vi "getAxisSignalQuality.vi"(0 "connection ID":refnum<k5>, 1 "axis":i32, 5 "error":errorcluster) -> (14 "connection ID out":refnum<k5>, 15 "axis_out":i32, 16 "contrast":i32, 17 "baseline":i32, 19 "error out":errorcluster)   [LabVIEW 2016, in "sen_api.lvlib"]
doc: "This function can be used to monitor the signal contrast (peak-to-peak of the basic interference signal amplitude) and the baseline (its offset) during a running measurement."
uses:
  sen_api.lvlib
panel:
  out "jsonRespIn":string
  out "JSON-response":string="{\"jsonrpc\":\"2.0\",\"method\":\"\",\"params\":[5,1.245,true,\"name\"],\"id\":\"1\"}"
  out "JSON request":string
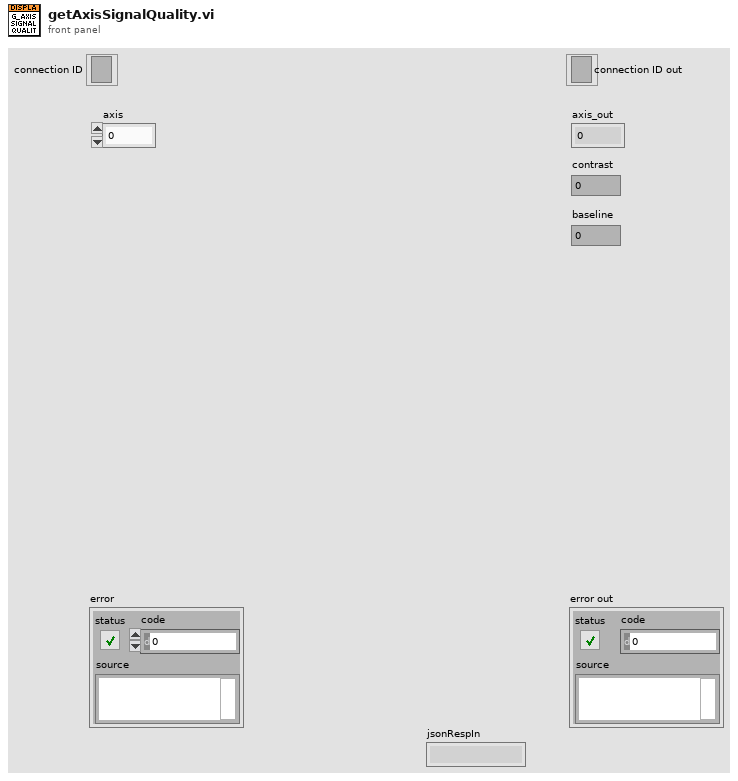
[diagram p1: front panel]
types:
  T1 = cluster{"jsonrpc":string, "method":string, "params":string[], "id":string, "api":i32, "pid":string}
  T2 = enum16{"Standard", "Buffered", "CRLF", "Immediate"}
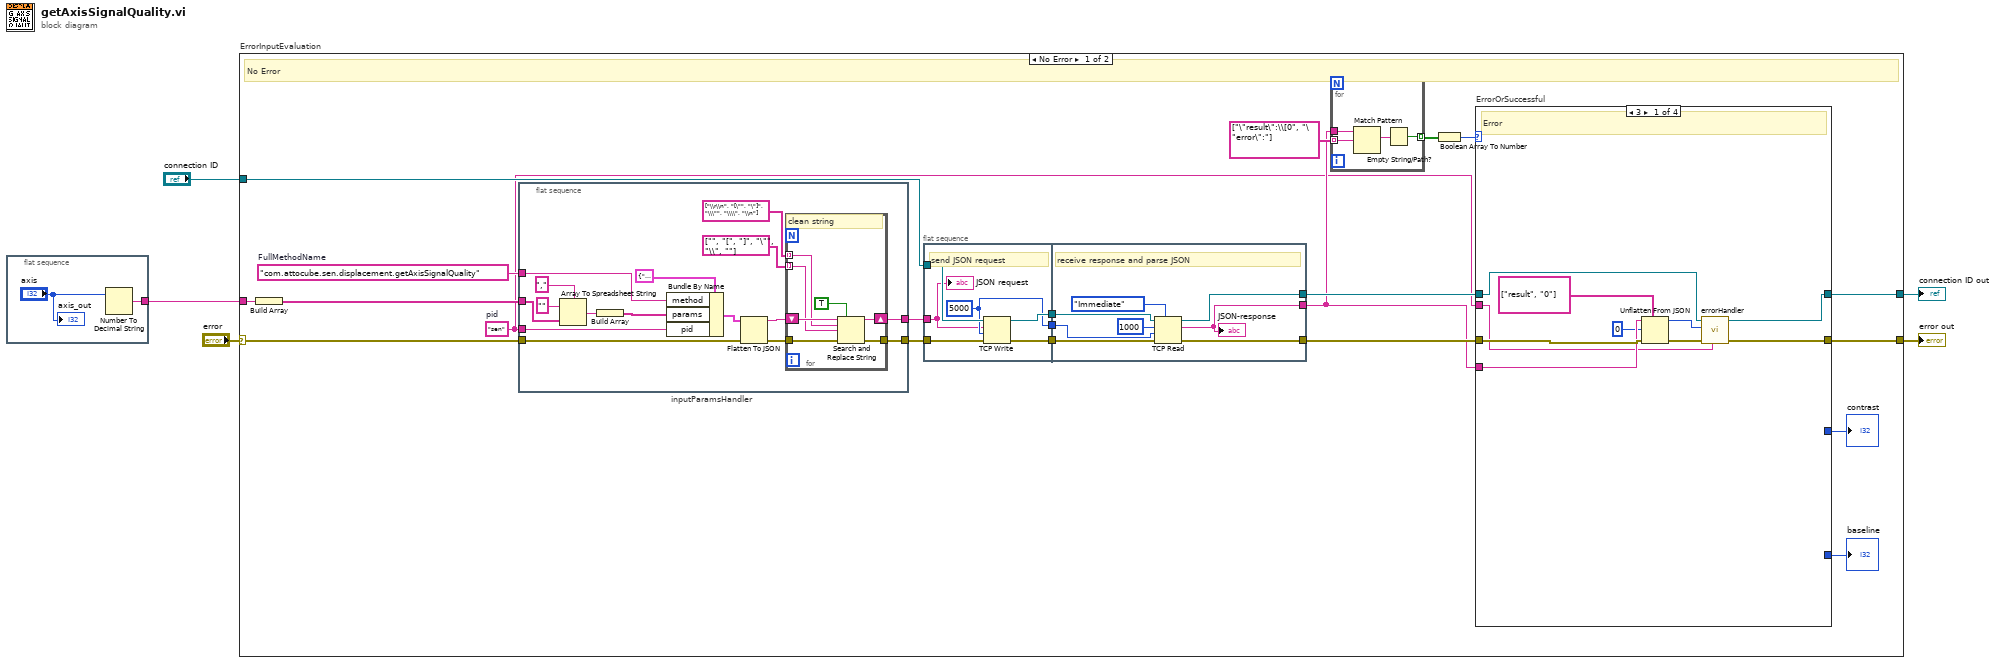
[diagram p0: block diagram]
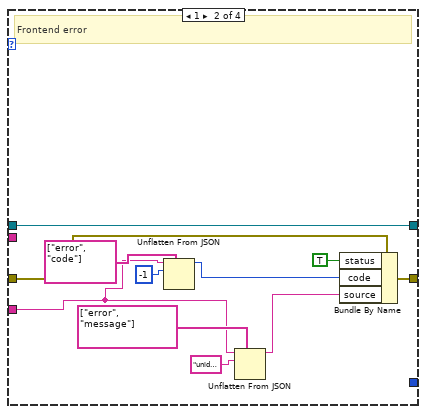
[diagram p2: hidden frame]
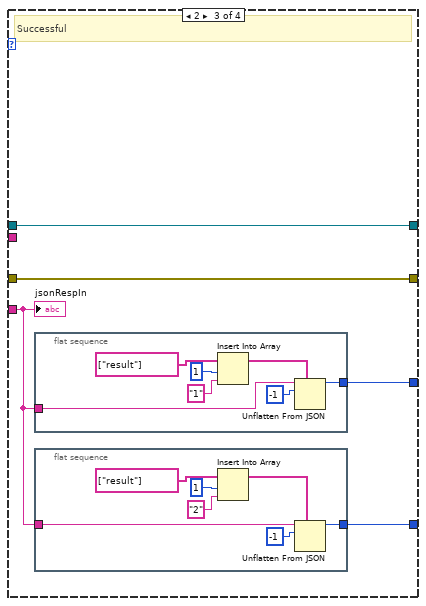
[diagram p3: hidden frame]
diagram:
  n1 = flat-sequence "in_axis" {
    tunnel: [w7] -> w1
    frame #0 {
      n2 = Number To Decimal String(number="axis") -> (decimal integer string=w7:string)  [unwired: 1 in]
      "axis_out" <- "axis"
    }
  }
  n3 = case "ErrorInputEvaluation" shown="No Error" "error" {
    selector: "error" -> [w21 w112]
    tunnel: "connection ID" -> [w25 w113]
    tunnel: [w12 w112] -> w4
    tunnel: [w13 w113] -> w3
    tunnel: w1 -> [w10 _]
    frame No Error {
      w11 = "sen"  # pid
      w22 = "com.attocube.sen.displacement.getAxisSignalQuality"  # FullMethodName
      # "No Error"
      n4 = Build Array ("ParametersArrayString")(w10) -> (w20:string[])
      n5 = flat-sequence "inputParamsHandler" {
        tunnel: [w74] -> w19
        tunnel: w20 -> [w81]
        tunnel: w21 -> [w79]
        tunnel: [w76] -> w18
        tunnel: w22 -> [w82]
        tunnel: w11 -> [w71]
        frame #0 {
          n6 = Array To Spreadsheet String(delimiter (Tab)=",", array=w81, 3:"" ("format string")) -> (spreadsheet string=w84:string)
          n7 = Build Array "Build Array"(w84) -> (w80:string[])
          n8 = Bundle By Name(cluster=T1 {"jsonrpc"="2.0", "method"="com.attocube.amc.res.setRESReadOutFreq", "params"=[], "id"="1", "api"=2, "pid"=""} ("Cluster"), "method"=w82, "params"=w80, "pid"=w71) -> (w83:T1)
          n9 = Flatten To JSON(anything=w83, error in (no error)=w79) -> (JSON string=w75:string, 11:w77:errorcluster)  [unwired: 1 in]
          n10 = for {
            tunnel: string[] ["\\r\\n", "[\"", "\"]", "\\\"", "\\\\", "\\n"] ("search string") -> [w90] mode=indexing
            tunnel: string[] ["", "[", "]", "\"", "\\", ""] ("replace string (\"\")") -> [w89] mode=indexing
            shift-right: [w92] -> w74
            shift-left: w75 -> [w91]
            tunnel: w77 -> [w88]
            tunnel: [w87] -> w76
            # "clean string"
            n11 = Search and Replace String(replace all?=TRUE ("replace all? (F)"), input string=w91, search string=w90, replace string=w89, error in=w88) -> (result string=w92:string, error out=w87:errorcluster)  [unwired: 3 in, 2 out]
          }
        }
      }
      n12 = flat-sequence {
        tunnel: w25 -> [w103]
        tunnel: [w101] -> w28
        tunnel: [w102] -> w27
        tunnel: w18 -> [w98]
        tunnel: [w100] -> w26
        tunnel: w19 -> [w99]
        tunnel: [w107] -> w17
        tunnel: w28 -> [w109]
        tunnel: w27 -> [w108]
        tunnel: [w105] -> w16
        tunnel: w26 -> [w106]
        tunnel: [w104] -> w15
        frame #0 {
          w100 = 5000 ("timeout ms (25000)")
          # "send JSON request"
          n13 = TCP Write(connection ID=w103, data in=w99, error in (no error)=w98, 9:w100) -> (connection ID out=w101:refnum<k5>, error out=w102:errorcluster)  [unwired: 1 out]
          "JSON request" <- w99
        }
        frame #1 {
          # "receive response and parse JSON"
          n14 = TCP Read(connection ID=w109, bytes to read=1000, error in (no error)=w108, 7:T2."Immediate" ("mode (standard)"), 9:w106) -> (connection ID out=w107:refnum<k5>, data out=w104:string, error out=w105:errorcluster)
          "JSON-response" <- w104
        }
      }
      n15 = for {
        tunnel: string[] ["\"result\":\\[0", "\"error\":"] ("path") -> [w96] mode=indexing
        tunnel: [w94] -> w23 mode=indexing
        tunnel: w15 -> [w97]
        n16 = Match Pattern(string=w97, regular expression=w96) -> (match substring=w95:string)  [unwired: 1 in, 3 out]
        n17 = Empty String/Path?(string/path=w95) -> (empty?=w94:bool)
      }
      n18 = Boolean Array To Number(Boolean array=w23) -> (number=w14:u32)
      n19 = case "ErrorOrSuccessful" shown="3" w14 {
        tunnel: w15 -> [w32 w41 w52 _]
        tunnel: w17 -> [w36 w39 w54 w70]
        tunnel: [w34 w39 w54 w70] -> w13
        tunnel: [w35 w42 w53 w69] -> w12
        tunnel: w16 -> [w38 w40 w53 w69]
        tunnel: w11 -> [w29 _ _ _]
        tunnel: [_ _ w51 _] -> w9
        tunnel: [_ _ w50 _] -> w8
        frame 3 {
          # "Error"
          n20 = Unflatten From JSON(path=string[] ["result", "0"], JSON string=w32, type and defaults=0, error in (no error)=w38) -> (value=w30:i32, error out=w37:errorcluster)  [unwired: 3 in]
          n21 = call "errorHandler.vi"("pid"=w29, "error in"=w37, "errNbr"=w30, "connection ID"=w36) -> ("error out 2"=w35:errorcluster, "connection ID out"=w34:refnum<k5>)  [unwired: 6 in]
        }
        frame 1 {
          # "Frontend error"
          n22 = Unflatten From JSON(path=string[] ["error", "code"], JSON string=w41, type and defaults=-1) -> (value=w48:i32)  [unwired: 4 in, 1 out]
          n23 = Unflatten From JSON(path=string[] ["error", "message"], JSON string=w41, type and defaults="unidentified error") -> (value=w49:string)  [unwired: 4 in, 1 out]
          n24 = Bundle By Name(cluster=w40, "status"=TRUE, "code"=w48, "source"=w49) -> (w42:errorcluster)
        }
        frame 2 {
          # "Successful"
          n25 = flat-sequence "out_integer" {
            tunnel: w52 -> [w64]
            tunnel: [w62] -> w51
            frame #0 {
              n26 = Insert Into Array(array=string[] ["result"] ("path"), index=1, new element="1" ("idx")) -> (w66:string[])
              n27 = Unflatten From JSON(path=w66, JSON string=w64, type and defaults=-1 ("index")) -> (value=w62:i32)  [unwired: 4 in, 1 out]
            }
          }
          n28 = flat-sequence "out_integer" {
            tunnel: w52 -> [w57]
            tunnel: [w55] -> w50
            frame #0 {
              n29 = Insert Into Array(array=string[] ["result"] ("path"), index=1, new element="2" ("idx")) -> (w59:string[])
              n30 = Unflatten From JSON(path=w59, JSON string=w57, type and defaults=-1 ("index")) -> (value=w55:i32)  [unwired: 4 in, 1 out]
            }
          }
          "jsonRespIn" <- w52
        }
        frame Default {
          # "NoResponse"
        }
      }
      "contrast" <- w9
      "baseline" <- w8
    }
    frame Error {
      # "Error"
    }
  }
  "error out" <- w4
  "connection ID out" <- w3
